vi "Wait_notification.vi"(10 "timeup":i32=-1, 11 "notification":i32) -> (3 "massage":string)   [LabVIEW 2011]
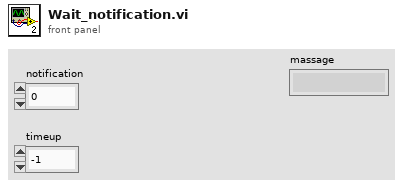
[diagram p1: front panel]
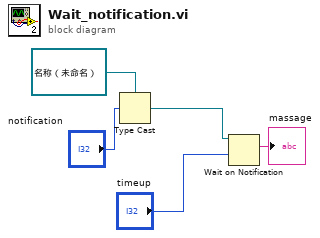
[diagram p0: block diagram]
diagram:
  n1 = Type Cast(type=refnum<notifier> refnum ("通知器输出"), x="notification") -> (*(type *) &x=w3:refnum<notifier>)
  n2 = Wait on Notification(notifier=w3, timeout in ms (-1)="timeup") -> (notification=→"massage":string)  [unwired: 2 in, 3 out]
